vi "Get_No_Top_Level_Message.vi"(11 "Build in":refnum<class "AB_PackedLibrary.lvclass">) -> (2 "No top level VI":string, 3 "Build out":refnum<class "AB_PackedLibrary.lvclass">)   [LabVIEW 2020, in "AB_PackedLibrary.lvclass"]
uses:
  <vilib>/AppBuilder/AB_Classes/PackedLib/AB_PackedLibrary.lvclass
  <resource>/Framework/Providers/Common/provcom_StringGlobals.vi
  <vilib>/AppBuilder/AB_Classes/PackedLib/AB_PackedLibrary.lvclass/AB_PackedLibrary.ctl
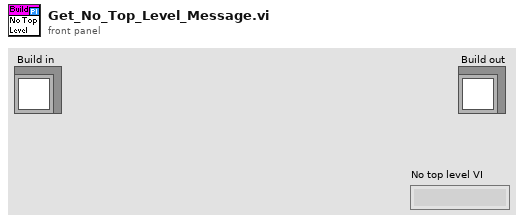
[diagram p1: front panel]
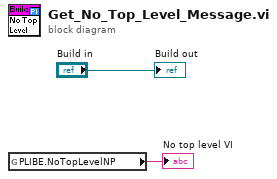
[diagram p0: block diagram]
diagram:
  n1 = global read "provcom_StringGlobals.vi" "PLIBE.NoTopLevelNP"() -> (→"No top level VI":string)
  "Build out" <- "Build in"
